vi "Get Config Data for Result Validation.vi"(8 "error in":errorcluster, 10 "GU Selected":i32[](array[numeric]), 11 "Config Data":T1(array[cluster])) -> (0 "error out":errorcluster, 1 "Number of GU":i32, 2 "Config Data":string[][](array[string]), 3 "Config Data dup":T1(array[cluster]), 4 "GU Numbers":string[](array[string]))   [LabVIEW 2020, in "GUCalibration2.lvlib"]
uses:
  GUCalibration2.lvlib
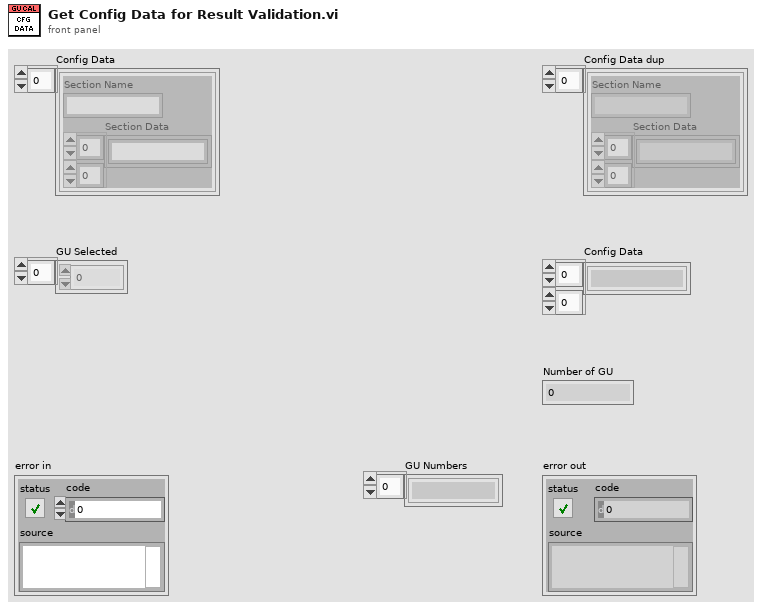
[diagram p1: front panel]
types:
  T1 = cluster{"Section Name":string, "Section Data":string[][]}[]
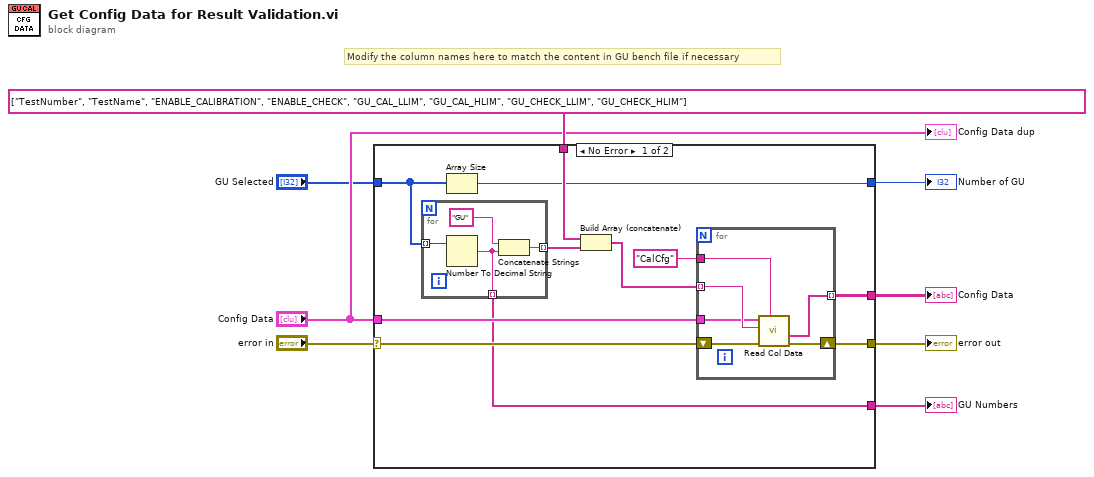
[diagram p0: block diagram]
diagram:
  # "Modify the column names here to match the content in GU bench file if necessary"
  n1 = case shown="No Error" "error in" {
    selector: "error in" -> [w19 w30]
    tunnel: "Config Data" -> [w18 _]
    tunnel: string[] ["TestNumber", "TestName", "ENABLE_CALIBRATION", "ENABLE_CHECK", "GU_CAL_LLIM", "GU_CAL_HLIM", "GU_CHECK_LLIM", "GU_CHECK_HLIM"] -> [w16 _]
    tunnel: [w15 _] -> w1
    tunnel: [w14 w30] -> w6
    tunnel: [w13 _] -> w4
    tunnel: [w11 _] -> w3
    tunnel: "GU Selected" -> [w10 _]
    frame No Error {
      n2 = for {
        tunnel: w10 -> [w22] mode=indexing
        tunnel: [w21] -> w12 mode=indexing
        tunnel: [w20] -> w11 mode=indexing
        n3 = Number To Decimal String(number=w22) -> (decimal integer string=w20:string)  [unwired: 1 in]
        n4 = Concatenate Strings("GU" ("element"), w20) -> (w21:string)
      }
      n5 = Array Size(array=w10) -> (size(s)=w13:i32)
      n6 = Build Array (concatenate)(w16, w12) -> (w9:string[])
      n7 = for {
        tunnel: w9 -> [w28] mode=indexing
        tunnel: "CalCfg" ("Section Name") -> [w27]
        shift-right: [w26] -> w14
        shift-left: w19 -> [w29]
        tunnel: [w25] -> w15 mode=indexing
        tunnel: w18 -> [w24]
        n8 = call "Read Col Data.vi"("Section Name"=w27, "error in (no error)"=w29, "Col Header Name"=w28, "Config Data"=w24) -> ("error out"=w26:errorcluster, "Column Data"=w25:string[])  [unwired: 4 in, 2 out]
      }
    }
    frame Error {
    }
  }
  "error out" <- w6
  "Config Data" <- w1
  "Number of GU" <- w4
  "GU Numbers" <- w3
  "Config Data dup" <- "Config Data"
